vi "GetRFrxCal.vi"(6 "Legacy (f)?":bool, 8 "error in (no error)":errorcluster, 10 "Freq Range":dbl[](array[numeric])) -> (0 "error out":errorcluster, 2 "Rx Cal Data":dbl[](array[numeric]))   [LabVIEW 2011]
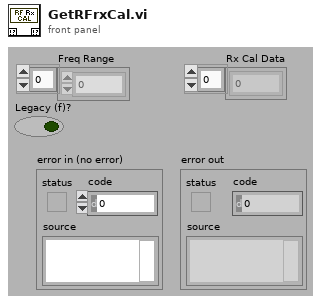
[diagram p1: front panel]
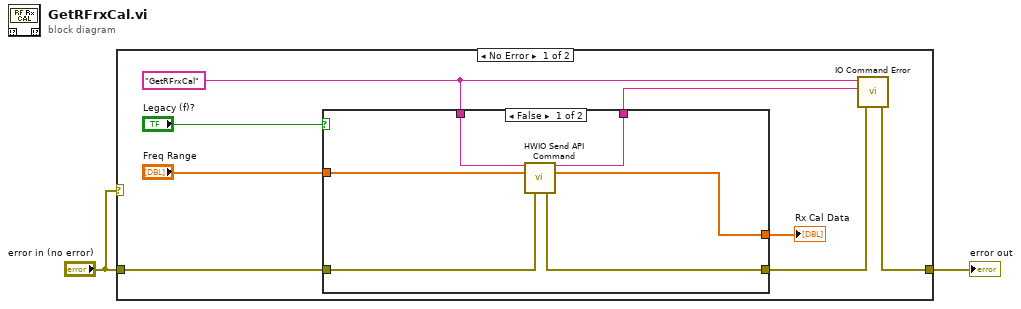
[diagram p0: block diagram]
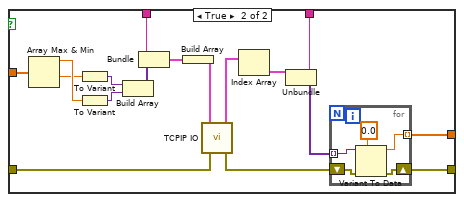
[diagram p2: hidden frame]
diagram:
  n1 = case shown="No Error" "error in (no error)" {
    tunnel: "error in (no error)" -> [w10 w39]
    tunnel: [w8 w39] -> w2
    frame No Error {
      w6 = "GetRFrxCal"
      n2 = case shown="False" "Legacy (f)?" {
        tunnel: w10 -> [w16 w32]
        tunnel: [w15 w30] -> w9
        tunnel: [w11 w29] -> w7
        tunnel: w6 -> [w12 w28]
        tunnel: "Freq Range" -> [w13 w21]
        tunnel: [w14 w17] -> w4
        frame False {
          n3 = call "HWIO Send API Command.vi"("Action"=w12, "Double"=w13, "error in (no error)"=w16) -> ("Action out"=w11:string, "Double out"=w14:dbl[], "error out"=w15:errorcluster)  [unwired: 5 in, 5 out]
        }
        frame True {
          n4 = Array Max & Min(array=w21) -> (max value=w20:dbl, min value=w19:dbl)  [unwired: 2 out]
          n5 = To Variant(anything=w19) -> (Variant=w24:variant)
          n6 = To Variant(anything=w20) -> (Variant=w22:variant)
          n7 = Build Array(w24, w22) -> (w23:variant[])
          n8 = Bundle(w28, w23) -> (w33:cluster{string, variant[]})  [unwired: 1 out]
          n9 = Build Array(w33) -> (w25:cluster{string, variant[]}[])
          n10 = call "TCPIP IO.vi"("error in (no error)"=w32, "Commands"=w25) -> ("error out"=w31:errorcluster, "Responses"=w27:cluster{string, variant[]}[])  [unwired: 1 in, 3 out]
          n11 = Index Array(array=w27) -> (element=w26:cluster{string, variant[]})  [unwired: 1 in]
          n12 = Unbundle(w26) -> (w29:string, w18:variant[])
          n13 = for {
            shift-right: [w37] -> w30
            shift-left: w31 -> [w38]
            tunnel: w18 -> [w35] mode=indexing
            tunnel: [w34] -> w17 mode=indexing
            n14 = Variant To Data(error in=w38, type=0.0 ("Injected Power, dBm"), Variant=w35) -> (data=w34:dbl, error out=w37:errorcluster)
          }
        }
      }
      "Rx Cal Data" <- w4
      n15 = call "IO Command Error.vi"("error in (no error)"=w9, "Command Returned (\"\")"=w7, "Command Sent (\"\")"=w6) -> ("error out"=w8:errorcluster)  [unwired: 4 out]
    }
    frame Error {
    }
  }
  "error out" <- w2
